vi "Set Named Range.vi"(7 "Sheet Name":string, 8 "error in":errorcluster, 9 "Cell Range":string="A1:B1", 10 "Named Range Identifier":string, 11 "SpreadsheetDoc in":refnum<k24>) -> (0 "error out":errorcluster, 3 "SpreadsheetDoc out":refnum<k24>)   [LabVIEW 2019, in "Open Xml.lvlib"]
uses:
  Open Xml.lvlib
  D:/git/Open-Xml-LabVIEW/Source/DocumentFormat.OpenXml.dll
  DocumentFormat.OpenXml.dll
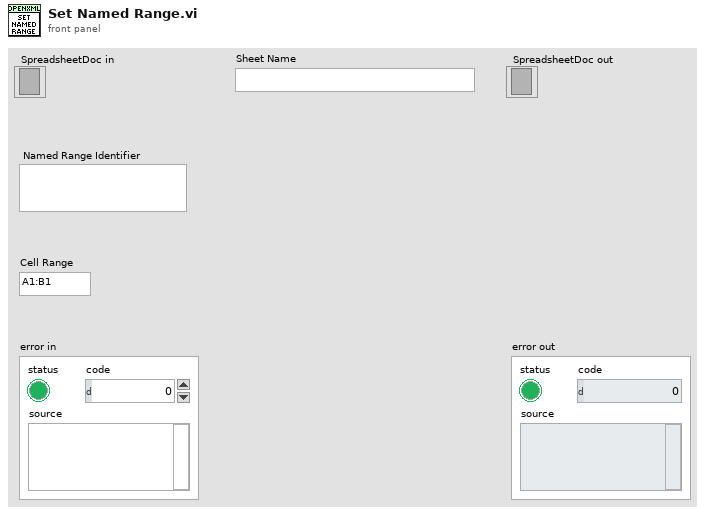
[diagram p1: front panel]
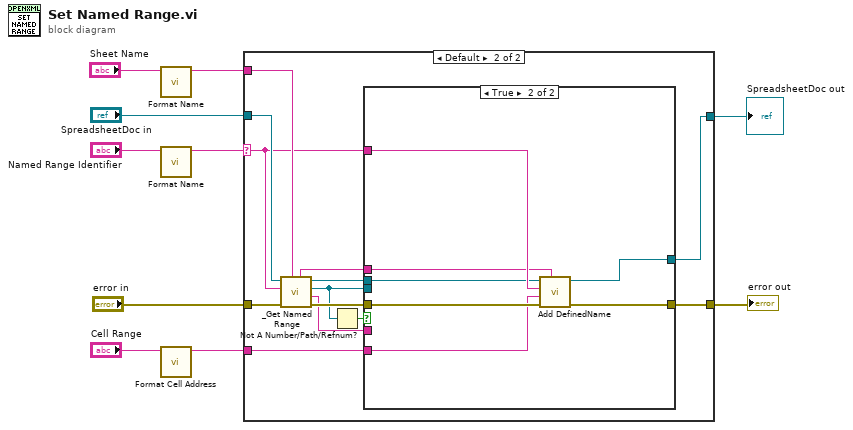
[diagram p0: block diagram]
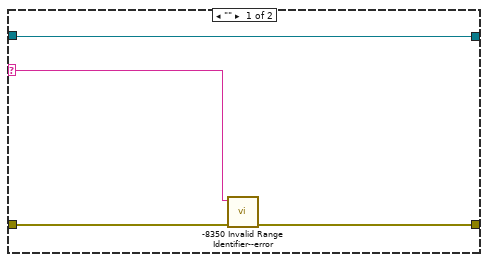
[diagram p2: hidden frame]
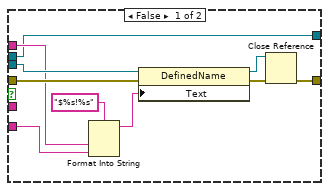
[diagram p3: hidden frame]
diagram:
  n1 = call "Format Name.vi"("Sheet Name"="Sheet Name") -> ("Formatted Sheet Name"=w3:string)  [unwired: 10 in]
  n2 = call "Format Name.vi"("Sheet Name"="Named Range Identifier") -> ("Formatted Sheet Name"=w2:string)  [unwired: 10 in]
  n3 = call "Format Cell Address.vi"("Cell Address"="Cell Range") -> ("Formatted Cell Address"=w1:string)  [unwired: 10 in]
  n4 = case shown="Default" w2 {
    selector: w2 -> [w12 w19]
    tunnel: "error in" -> [w14 w27]
    tunnel: [w13 w24] -> w4
    tunnel: "SpreadsheetDoc in" -> [w11 w25]
    tunnel: [w11 w17] -> w9
    tunnel: w3 -> [_ w23]
    tunnel: w1 -> [_ w18]
    frame "" {
      n5 = call "-8350 Invalid Range Identifier--error.vi"("error in"=w14, "Argument"=w12) -> ("error out"=w13:errorcluster)  [unwired: 9 in]
    }
    frame Default {
      n6 = call "_Get Named Range.vi"("Sheet Name"=w23, "error in"=w27, "Range Identifier"=w19, "SpreadsheetDoc in"=w25) -> ("error out"=w26:errorcluster, "Range"=w16:string, "DefinedName"=w15:refnum<k24>, "SpreadsheetDoc out"=w21:refnum<k24>, "Sheet Name"=w22:string)  [unwired: 3 in]
      n7 = Not A Number/Path/Refnum?(number/path/refnum=w15) -> (NaN/Path/Refnum?=w20:bool)
      n8 = case shown="True" w20 {
        tunnel: w26 -> [w37 w44]
        tunnel: w21 -> [w28 w40]
        tunnel: [w30 w43] -> w24
        tunnel: w22 -> [w32 w39]
        tunnel: w19 -> [_ w42]
        tunnel: w18 -> [w31 w41]
        tunnel: [w28 w38] -> w17
        tunnel: w16 -> [_ _]
        tunnel: w15 -> [w35 _]
        frame False {
          n9 = Format Into String(format string="$%s!%s", w32, w31) -> (resulting string=w34:string)  [unwired: 2 in, 1 out]
          n10 = property class="DefinedName"(reference=w35, error in=w37, "Text"=w34) -> (reference out=w29:refnum<k24>, error out=w36:errorcluster)
          n11 = Close Reference(reference=w29, error in (no error)=w36) -> (error out=w30:errorcluster)
        }
        frame True {
          n12 = call "Add DefinedName.vi"("Sheet Name"=w39, "error in"=w44, "Cell Range"=w41, "Identifier"=w42, "SpreadsheetDoc in"=w40) -> ("error out"=w43:errorcluster, "SpreadsheetDoc out"=w38:refnum<k24>)  [unwired: 5 in]
        }
      }
    }
  }
  "SpreadsheetDoc out" <- w9
  "error out" <- w4
